vi "Init.vi"(8 "error in (no error)":errorcluster, 10 "ICameraTesting":refnum<class "ICameraTesting.lvclass">, 11 "CameraTestingENI":refnum<class "CameraTestingENI.lvclass">) -> (0 "error out":errorcluster, 3 "CameraTestingENI":refnum<class "CameraTestingENI.lvclass">)   [LabVIEW 2020, in "CameraTestingProxy.lvlib" / "CameraTestingENI.lvclass"]
uses:
  CameraTestingENI.lvclass
  E:/GitHub/Evaluation_Test/Labview/src/CameraTestingApp/ICameraTestingUI/ICameraTestingUI/ICameraTestingUI.lvclass
  CameraTestingApp/ICameraTesting/ICameraTesting/ICameraTesting.lvclass
  Private/TypeDef/InitMsgStates.ctl
  CameraTestingENI.lvclass/CameraTestingENI.ctl
  <vilib>/ActorFramework/Message Enqueuer/Message Enqueuer.lvclass/Message Enqueuer.ctl
  <vilib>/ActorFramework/Message Enqueuer/Message Priority.ctl
  <vilib>/ActorFramework/Message Enqueuer/Enqueue.vi
  CameraTestingApp/ICameraTesting/ICameraTesting Messages/AcqVideoOptCodes Msg/AcqVideoOptCodes Msg.lvclass
  C:/Program Files (x86)/National Instruments/LabVIEW 2020/vi.lib/ActorFramework/Message/Message.lvclass
  CameraTestingApp/ICameraTesting/ICameraTesting Messages/GetEvents Msg/GetEvents Msg.lvclass
  <vilib>/ActorFramework/Message Priority Queue/Priority Enqueue.vi
  <vilib>/ActorFramework/Message Enqueuer/Message Enqueuer.lvclass
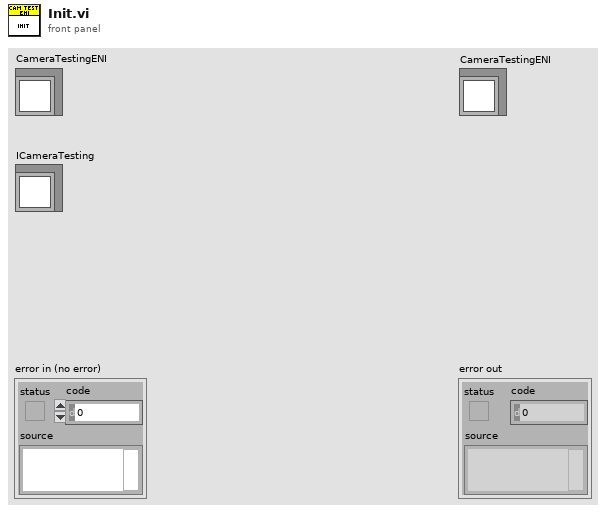
[diagram p1: front panel]
types:
  T1 = typedef "CameraTestingProxy.lvlib/CameraTestingENI.lvclass/InitMsgStates.ctl" = enum16{"Launch Controller", "Request Video Options Values", "Get CameraTesting Evenrs"}
  T2 = typedef "Actor Framework.lvlib/Message Enqueuer.lvclass/Message Priority.ctl" = enum16{"Low", "Normal", "High"}
  T3 = typedef "CameraTestingProxy.lvlib/CameraTestingENI.lvclass/CamTestEnqrReceived.ctl" = refnum<user-event>
  T4 = typedef "ICameraTesting_typedef.lvlib/CameraInfo.ctl" = cluster{"ICamera ":refnum<class "ICamera.lvclass">, "Connection String":string}
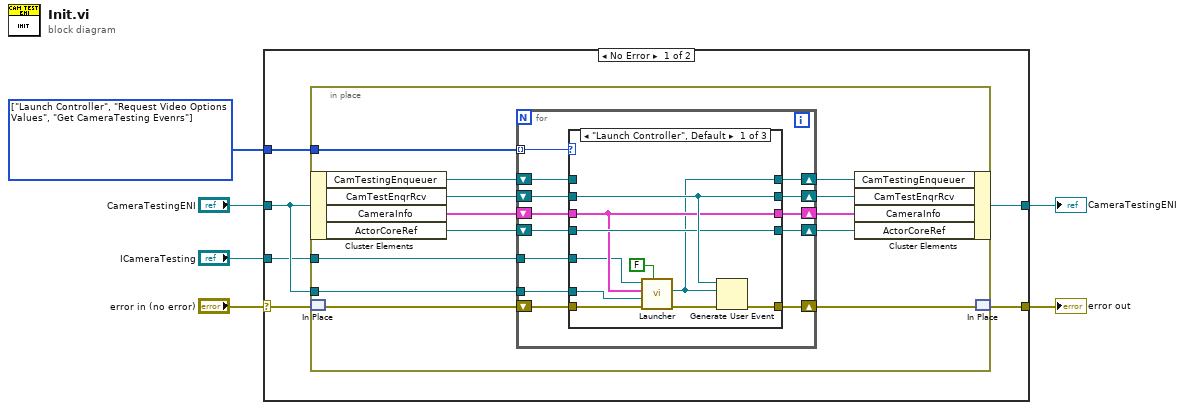
[diagram p0: block diagram]
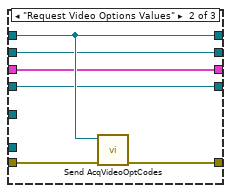
[diagram p2: hidden frame]
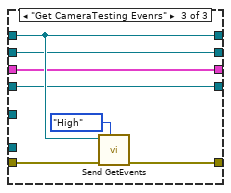
[diagram p3: hidden frame]
diagram:
  w2 = T1[] [enum."Launch Controller", enum."Request Video Options Values", enum."Get CameraTesting Evenrs"] items=["Launch Controller", "Request Video Options Values", "Get CameraTesting Evenrs"]
  n1 = case shown="No Error" "error in (no error)" {
    selector: "error in (no error)" -> [w11 w63]
    tunnel: [w10 w63] -> w5
    tunnel: [w9 w62] -> w3
    tunnel: "CameraTestingENI" -> [w8 w62]
    tunnel: w2 -> [w12 _]
    tunnel: "ICameraTesting" -> [w7 _]
    frame No Error {
      n2 = in-place {
        in-place-border: w12 -> [w25]
        in-place-border: w8 -> [w15]
        in-place-border: w7 -> [w13]
        n3 = in-place-cluster #1(w8) -> ("CamTestingEnqueuer"=w22:refnum<class "Message Enqueuer.lvclass">, "CamTestEnqrRcv"=w21:T3, "CameraInfo"=w20:T4, "ActorCoreRef"=w19:refnum<vi>)
        n4 = in-place-match #2(w11) -> (w24:errorcluster)
        n5 = for {
          shift-right: [w37] -> w23
          shift-left: w24 -> [w38]
          tunnel: w25 -> [w36] mode=indexing
          shift-right: [w27] -> w16
          shift-left: w19 -> [w28]
          shift-right: [w30] -> w14
          shift-left: w20 -> [w31]
          shift-right: [w32] -> w17
          shift-left: w21 -> [w33]
          shift-right: [w34] -> w18
          shift-left: w22 -> [w35]
          tunnel: w15 -> [w29]
          tunnel: w13 -> [w26]
          n6 = case shown="\"Launch Controller\", Default" w36 {
            tunnel: w38 -> [w44 w54 w60]
            tunnel: [w48 w53 w55] -> w37
            tunnel: w35 -> [_ w52 w59]
            tunnel: [w39 w52 w59] -> w34
            tunnel: w33 -> [w47 w51 w57]
            tunnel: [w47 w51 w57] -> w32
            tunnel: w31 -> [w41 w50 w56]
            tunnel: [w41 w50 w56] -> w30
            tunnel: w29 -> [w43 _ _]
            tunnel: w28 -> [w46 w49 w58]
            tunnel: [w46 w49 w58] -> w27
            tunnel: w26 -> [w40 _ _]
            frame "Launch Controller", Default {
              n7 = call-dynamic "Launcher.vi"("Open FP?"=FALSE, "error in (no error)"=w44, "ICameraTestingUI"=w43, "CameraInfo"=w41, "ICameraTesting in"=w40) -> ("error out"=w45:errorcluster, "CameraTesting Enqueuer"=w39:refnum<class "Message Enqueuer.lvclass">)  [unwired: 5 in]
              n8 = Generate User Event(user event=w47, event data cluster=w39, error in=w45) -> (error out=w48:errorcluster)  [unwired: 1 in, 1 out]
            }
            frame "Request Video Options Values" {
              n9 = call "Send AcqVideoOptCodes.vi"("error in (no error)"=w54, "Message Enqueuer"=w52) -> ("error out"=w53:errorcluster)  [unwired: 8 in, 1 out]
            }
            frame "Get CameraTesting Evenrs" {
              n10 = call "Send GetEvents.vi"("Message Priority (Normal)"=Message_Priority."High", "error in (no error)"=w60, "Message Enqueuer"=w59) -> ("error out"=w55:errorcluster)  [unwired: 7 in, 1 out]
            }
          }
        }
        n11 = in-place-cluster #1("CamTestingEnqueuer"=w18, "CamTestEnqrRcv"=w17, "CameraInfo"=w14, "ActorCoreRef"=w16) -> (w9:refnum<class "CameraTestingENI.lvclass">)
        n12 = in-place-match #2(w23) -> (w10:errorcluster)
      }
    }
    frame Error {
    }
  }
  "error out" <- w5
  "CameraTestingENI" <- w3
